vi "Poly_ReadAnalogIn.vi"   [LabVIEW 2012]
doc: "Reads the value of the specified analog \"Channel\" and returns that value as \"Variable Out\"."
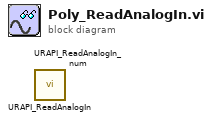
[diagram p0: block diagram]
diagram:
  n1 = call <userlib>:"URAPI_ReadAnalogIn.vi"() -> ()  [unwired: 4 in, 2 out]
  n2 = call <userlib>:"URAPI_ReadAnalogIn_num.vi"() -> ()  [unwired: 4 in, 2 out]
